vi "Test Decompose and Recompose.vi"() -> ()   [LabVIEW 2023]
uses:
  CTLs/Resource.ctl
  SubVIs/Decompose VI (Refnum).vi
panel:
  out "Target path out":path
  out "VI Load Result":errorcluster
  out "array of clusters":T2(array[cluster])
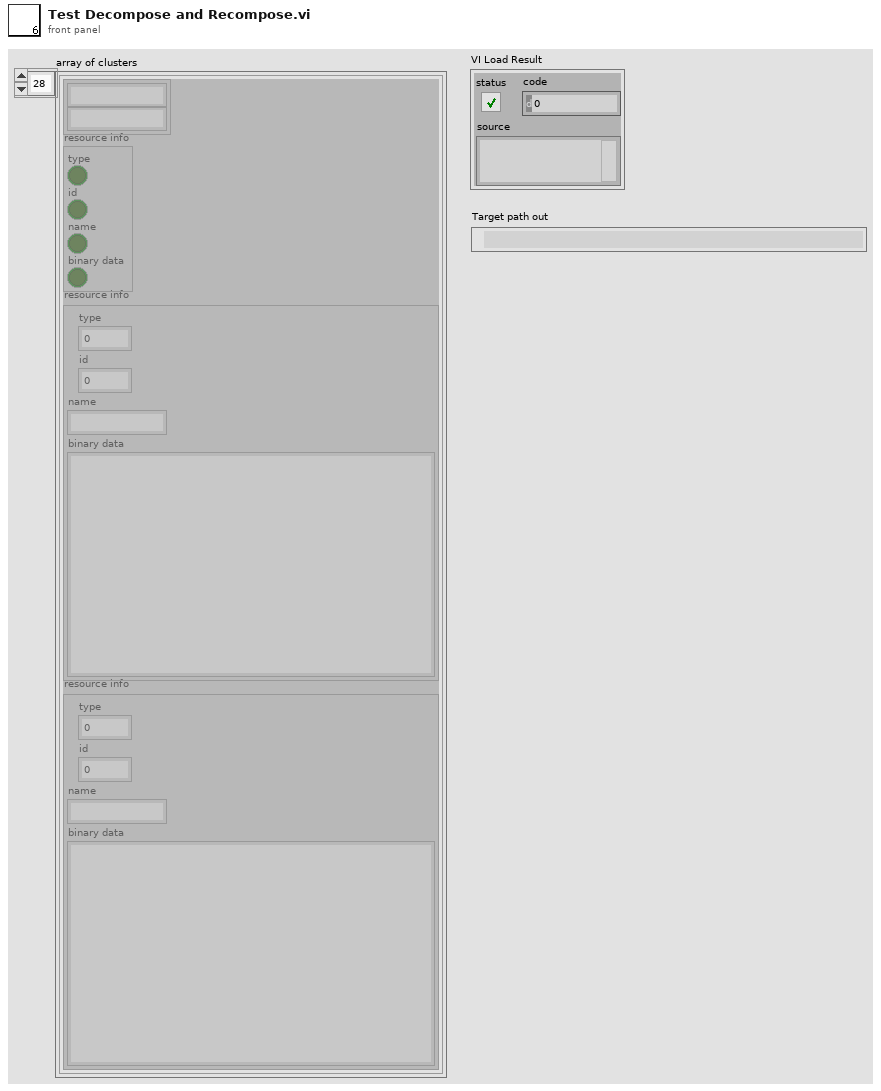
[diagram p1: front panel]
types:
  T1 = typedef "Resource.ctl" = cluster{"type":u32, "id":i32, "name":string, "binary data":string}
  T2 = cluster{cluster{string, string}, "resource info":cluster{"type":bool, "id":bool, "name":bool, "binary data":bool}, "resource info":T1, "resource info":T1}[]
  T3 = typedef "Resource Array.ctl" = T1[]
  T4 = cluster{"type":bool, "id":bool, "name":bool, "binary data":bool}[]
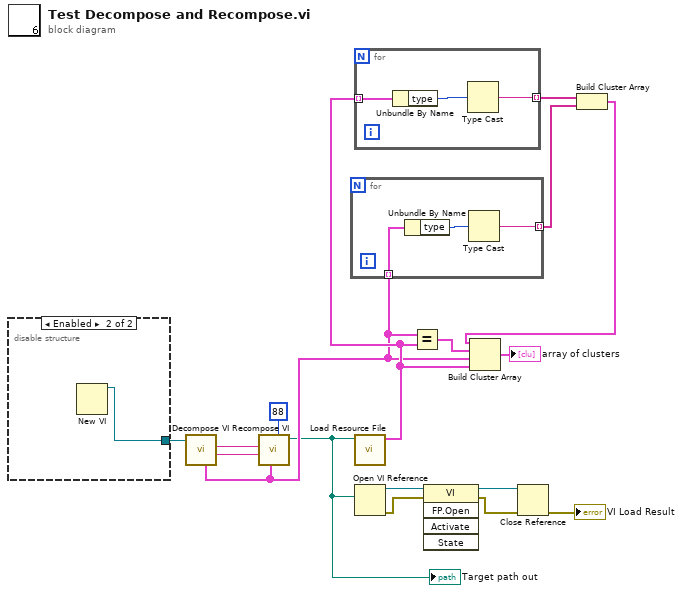
[diagram p0: block diagram]
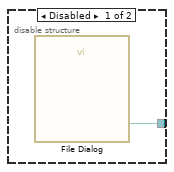
[diagram p2: hidden frame]
diagram:
  n1 = disable-structure shown="Enabled" {
    disable-tunnel: [w18 w19] -> w15
    frame Disabled {
      n2 = call "File Dialog"() -> ("selected path"=w18:path)  [unwired: 12 in, 3 out]
    }
    frame Enabled {
      n3 = New VI() -> (3:w19:refnum<vi>)  [unwired: 7 in, 1 out]
    }
  }
  n4 = call-poly "Decompose VI.vi"("VI Refnum"=w15) -> ("Block Diagram XML"=w17:string, "Front Panel XML"=w1:string, "Other resources"=w8:T3)  [unwired: 6 in, 2 out]
  n5 = call "Recompose VI.vi"("FPH_/BDH_ (88=X)"=u8 88, "Other resources (default)"=w8, "Block Diagram XML"=w17, "Front Panel XML"=w1) -> ("Target path out"=w7:path)  [unwired: 5 in, 2 out]
  "Target path out" <- w7
  n6 = for {
    tunnel: w8 -> [w22] mode=indexing
    tunnel: [w20] -> w11 mode=indexing
    n7 = Unbundle By Name(w22) -> ("type"=w21:u32)
    n8 = Type Cast(x=w21) -> (*(type *) &x=w20:string)  [unwired: 1 in]
  }
  n9 = call "Load Resource File.vi"("Resource File"=w7) -> ("Resources"=w13:T3)  [unwired: 8 in, 2 out]
  n10 = for {
    tunnel: w13 -> [w25] mode=indexing
    tunnel: [w23] -> w12 mode=indexing
    n11 = Unbundle By Name(w25) -> ("type"=w24:u32)
    n12 = Type Cast(x=w24) -> (*(type *) &x=w23:string)  [unwired: 1 in]
  }
  n13 = Open VI Reference(vi path=w7) -> (vi reference=w6:refnum<vi>, error out=w5:errorcluster)  [unwired: 5 in]
  n14 = Equal?(x=w8, y=w13) -> (x = y?=w14:T4)
  n15 = invoke class="VI" method="FP.Open"(reference=w6, error in=w5) -> (reference out=w4:refnum<vi>, error out=w3:errorcluster)  [unwired: 3 in, 3 out]
  n16 = Close Reference(reference=w4, error in (no error)=w3) -> (error out=→"VI Load Result":errorcluster)
  n17 = Build Cluster Array(w12, w11) -> (w10:cluster{string, string}[])
  n18 = Build Cluster Array(w10, w14, w8, w13) -> (→"array of clusters":T2)
